vi "Climb Deploy Level 1.vi"(10 "Command":T4, 11 "ServoDeviceRef":T1={"DeviceStatus"={"status"=FALSE, "code"=0, "source"=""}, "PWM Channel"=enum."Invalid", "DeadBand"={"Name"="", "maxPositivePwm"=0, "minPositivePwm"=0, "centerPwm"=0, "maxNegativePwm"=0, "minNegativePwm"=0, "angularRange"=0}}) -> (3 "Servo Output":dbl)   [LabVIEW 2017]
uses:
  <userlib>/836-Library/System/QCP_V2/QCPSupportCode/QCP_GetDbl.vi
  Climb Deploy.ctl
  <vilib>/Rock Robotics/SystemInterfaces/DIO/FPGA_DIOPWMChannel.ctl
  <vilib>/Rock Robotics/WPI/PWM/WPI_PWMDeadband.ctl
  <vilib>/Rock Robotics/WPI/PWM/Servo/WPI_ServoDeviceRef.ctl
panel:
  in  "Tuning Value":dbl
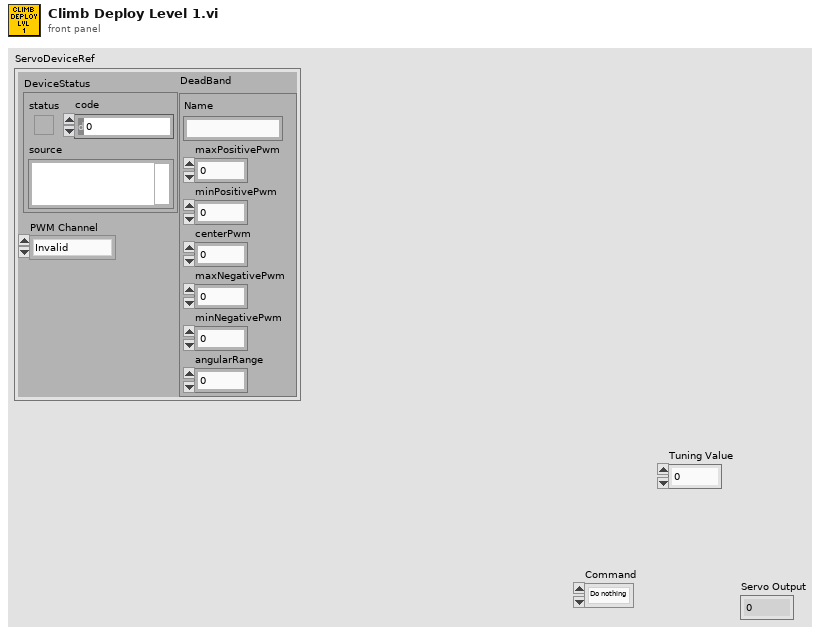
[diagram p1: front panel]
types:
  T1 = typedef "WPI_ServoDeviceRef.ctl" = cluster{"DeviceStatus":errorcluster, "PWM Channel":T2, "DeadBand":T3}
  T2 = typedef "FPGA_DIOPWMChannel.ctl" = enum8{"PWM 0", "PWM 1", "PWM 2", "PWM 3", "PWM 4", "PWM 5", "PWM 6", "PWM 7", "PWM 8", "PWM 9", "PWM MXP 0", "PWM MXP 1", "PWM MXP 2", "PWM MXP 3", "PWM MXP 4", "PWM MXP 5", "PWM MXP 6", "PWM MXP 7", "PWM MXP 8", "PWM MXP 9", "Invalid"}
  T3 = typedef "WPI_PWMDeadband.ctl" = cluster{"Name":string, "maxPositivePwm":i32, "minPositivePwm":i32, "centerPwm":i32, "maxNegativePwm":i32, "minNegativePwm":i32, "angularRange":u16}
  T4 = typedef "Climb Deploy.ctl" = enum16{"Do nothing", "Deploy"}
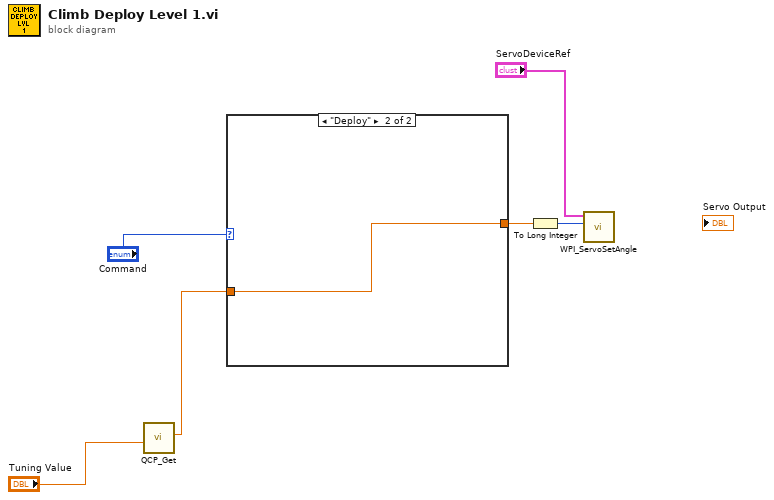
[diagram p0: block diagram]
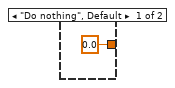
[diagram p2: hidden frame]
diagram:
  n1 = call-poly <userlib>:"QCP_Get.vi"("Tuning Value"="Tuning Value") -> ("Value"=w5:dbl)  [unwired: 8 in, 2 out]
  n2 = case shown="\"Deploy\"" "Command" {
    tunnel: w5 -> [_ w8]
    tunnel: [0.0 ("Value") w8] -> w3
    frame "Do nothing", Default {
    }
    frame "Deploy" {
    }
  }
  n3 = To Long Integer(number=w3) -> (32bit integer=w2:i32)
  n4 = call <vilib>:"WPI_ServoSetAngle.vi"("Angle"=w2, "ServoDeviceRef"="ServoDeviceRef") -> ()  [unwired: 8 in, 2 out]
